vi "Vector Field Histogram.vi"(4 "maximum heading change (rad)":dbl=1.5707963267948966, 5 "obstacle clearance distance":dbl, 6 "# bins":i32=399, 7 "heading":T1, 8 "error in (no error)":errorcluster, 9 "thresholds":T2, 10 "direction angles (rad)":dbl[](array[numeric]), 11 "distances":dbl[](array[numeric])) -> (0 "error out":errorcluster, 1 "mask":bool[](array[boolean]), 2 "histogram":dbl[](array[numeric]), 3 "chosen heading (rad)":dbl)   [LabVIEW 2017, in "NI_Robotics_Vector Field Histogram.lvlib"]
doc: "Identifies obstacles and gaps, or open areas, in the robot environment and returns an open direction for travel that best leads to a goal position."
uses:
  <vilib>/robotics/Obstacle Avoidance/Advanced Vector Field Histogram/NI_Robotics_Vector Field Histogram.lvlib
  <vilib>/robotics/Obstacle Avoidance/Advanced Vector Field Histogram/VFH Compute Config Space Range.vi
  <vilib>/robotics/Obstacle Avoidance/Advanced Vector Field Histogram/VFH Cost Function.vi
  <vilib>/Analysis/coordinate.llb/Wrap Angle.vi
  <vilib>/Analysis/coordinate.llb/Wrap Angle (scalar).vi
  <vilib>/robotics/Utilities/NI_Robotics Utilities.lvlib
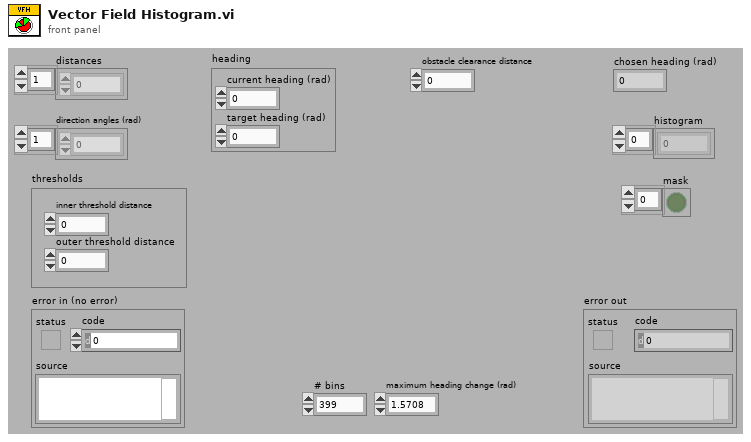
[diagram p1: front panel]
types:
  T1 = cluster{"current heading (rad)":dbl, "target heading (rad)":dbl}
  T2 = cluster{"inner threshold distance":dbl, "outer threshold distance":dbl}
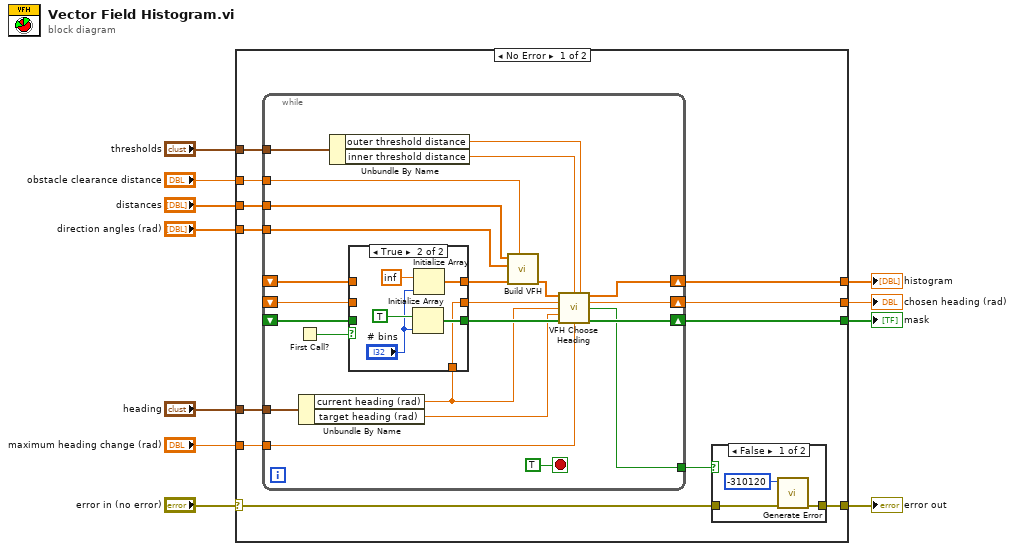
[diagram p0: block diagram]
diagram:
  n1 = case shown="No Error" "error in (no error)" {
    selector: "error in (no error)" -> [w12 w59]
    tunnel: "maximum heading change (rad)" -> [w23 _]
    tunnel: [w22 _] -> w10
    tunnel: "obstacle clearance distance" -> [w21 _]
    tunnel: [w20 _] -> w8
    tunnel: "distances" -> [w19 _]
    tunnel: "direction angles (rad)" -> [w18 _]
    tunnel: [w17 _] -> w5
    tunnel: "thresholds" -> [w16 _]
    tunnel: "heading" -> [w15 _]
    tunnel: [w13 w59] -> w1
    frame No Error {
      n2 = while {
        tunnel: w18 -> [w49]
        tunnel: w19 -> [w48]
        tunnel: [w35] -> w14
        tunnel: w23 -> [w45]
        tunnel: w21 -> [w42]
        shift-right: [w43] -> w22
        shift-left: _ -> [w41]
        shift-right: [w46] -> w17
        shift-left: _ -> [w39]
        shift-right: [w47] -> w20
        shift-left: _ -> [w40]
        tunnel: w16 -> [w34]
        tunnel: w15 -> [w30]
        stop <- TRUE stop-if-true
        n3 = First Call?() -> (First Call?: T/F=w28:bool)
        n4 = Unbundle By Name(w30) -> ("current heading (rad)"=w31:dbl, "target heading (rad)"=w29:dbl)
        n5 = Unbundle By Name(w34) -> ("outer threshold distance"=w33:dbl, "inner threshold distance"=w32:dbl)
        n6 = case shown="True" w28 {
          tunnel: w41 -> [w52 _]
          tunnel: w40 -> [w51 _]
          tunnel: w39 -> [w50 _]
          tunnel: [w52 w55] -> w38
          tunnel: [w51 w53] -> w37
          tunnel: [w50 w54] -> w36
          tunnel: w31 -> [_ w53]
          frame False {
          }
          frame True {
            n7 = Initialize Array(TRUE, "# bins") -> (w54:bool[])
            n8 = Initialize Array(inf ("element"), "# bins") -> (w55:dbl[])
          }
        }
        n9 = call <vilib>:"Build VFH.vi"("obstacle clearance (distance)"=w42, "histogram in"=w38, "sensor angles (radians)"=w49, "sensor range (distance)"=w48) -> ("histogram out"=w43:dbl[])  [unwired: 7 in]
        n10 = call <vilib>:"VFH Choose Heading.vi"("histogram in"=w43, "inner visibility threshold"=w32, "outer visibility threshold"=w33, "last commanded heading (rad)"=w37, "current heading (rad)"=w31, "target heading (rad)"=w29, "mask in"=w36, "maximum heading change (rad)"=w45) -> ("chosen heading (rad)"=w47:dbl, "heading found?"=w35:bool, "mask out"=w46:bool[])  [unwired: 5 in]
      }
      n11 = case shown="False" w14 {
        tunnel: [w25 w27] -> w13
        tunnel: w12 -> [w24 w27]
        frame False {
          n12 = call <vilib>:"Generate Error.vi"("error in (no error)"=w24, "code"=-310120) -> ("error out"=w25:errorcluster)  [unwired: 9 in]
        }
        frame True {
        }
      }
    }
    frame Error {
    }
  }
  "histogram" <- w10
  "chosen heading (rad)" <- w8
  "mask" <- w5
  "error out" <- w1
